vi "contrast move V0.5.vi"(8 "error in (no error)":errorcluster, 9 "Position in":T1, 11 "Target position":cluster{"X":dbl, "Y":dbl, "speed":dbl}) -> (0 "error out":errorcluster, 1 "Position out":T1)   [LabVIEW 2019]
uses:
  position cluster.ctl
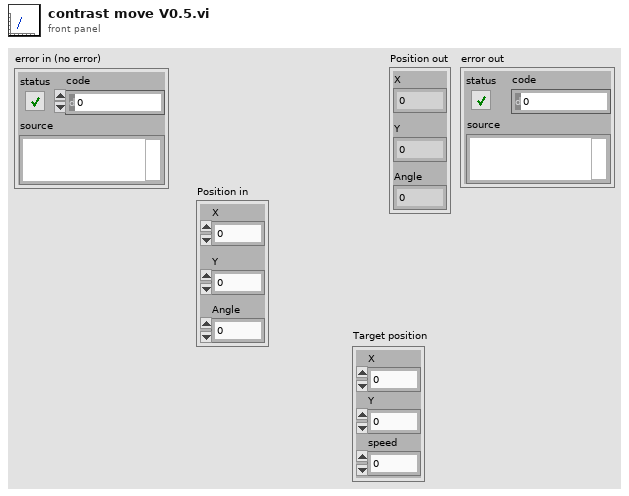
[diagram p1: front panel]
types:
  T1 = typedef "position cluster.ctl" = cluster{"X":dbl, "Y":dbl, "Angle":dbl}
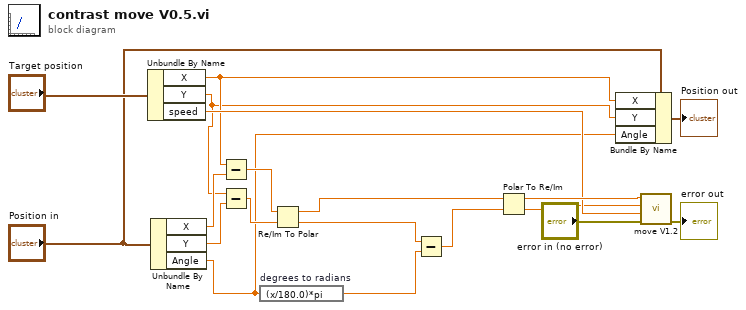
[diagram p0: block diagram]
diagram:
  n1 = Unbundle By Name("Target position") -> ("X"=w8:dbl, "Y"=w7:dbl, "speed"=w11:dbl)
  n2 = Unbundle By Name("Position in") -> ("X"=w13:dbl, "Y"=w12:dbl, "Angle"=w4:dbl)
  n3 = Subtract(x=w8, y=w13) -> (x-y=w14:dbl)
  n4 = Subtract(x=w7, y=w12) -> (x-y=w15:dbl)
  n5 = expression code="(x/180.0)*pi" "degrees to radians"(w4) -> (w3:dbl)
  n6 = Re/Im To Polar(2:w15, 3:w14) -> (0:w2:dbl, 1:w19:dbl)
  n7 = Subtract(x=w2, y=w3) -> (x-y=w18:dbl)
  n8 = Polar To Re/Im(2:w18, 3:w19) -> (0:w10:dbl, 1:w17:dbl)
  n9 = Bundle By Name(cluster="Position in", "X"=w8, "Y"=w7, "Angle"=w4) -> (→"Position out":T1)
  n10 = call "move V1.2.vi"("error in (no error)"="error in (no error)", "RPM"=w11, "Y"=w10, "X"=w17) -> ("error out"=→"error out":errorcluster)  [unwired: 7 in]
